vi "Handle Error.vi"(8 "error in (no error)":errorcluster, 11 "Measurement in":refnum<class "Measurement.lvclass">) -> (0 "error out":errorcluster, 2 "stop actor?":bool=TRUE, 3 "Measurement out":refnum<class "Measurement.lvclass">)   [LabVIEW 2015, in "Measurement Actor.lvlib" / "Measurement.lvclass"]
doc: "(<B>Filename</B>: Actor Framework.lvlib:Actor.lvclass:Handle Error.vi)\n\nDefines how the actor handles an error that occurred while processing a message.\n\nBy default, this method does nothing except stop the actor. This method also treats error code 43 (coming from <B>error in</B>) as a sign that the actor shut down normally. In this situation, the Handle Error method does not return the error on <B>error out</B>, meaning the actor's caller will not receive it. All other error codes will be returned on <B>error out</B>.\n\nA descendant class may override this method to change this behavior."
uses:
  Measurement.lvclass
  <vilib>/ActorFramework/Actor/Actor.lvclass/Actor.ctl
  <vilib>/ActorFramework/Actor/Actor.lvclass
  Controller/Messages/Log Status/Log Status.lvclass
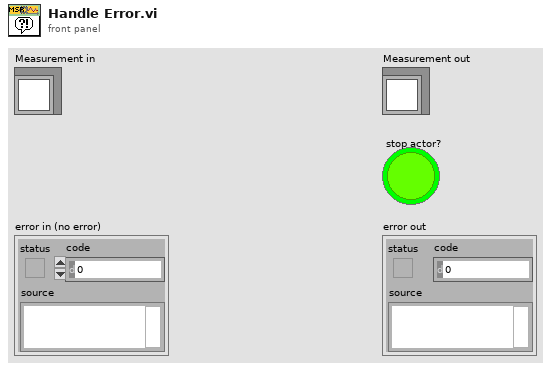
[diagram p1: front panel]
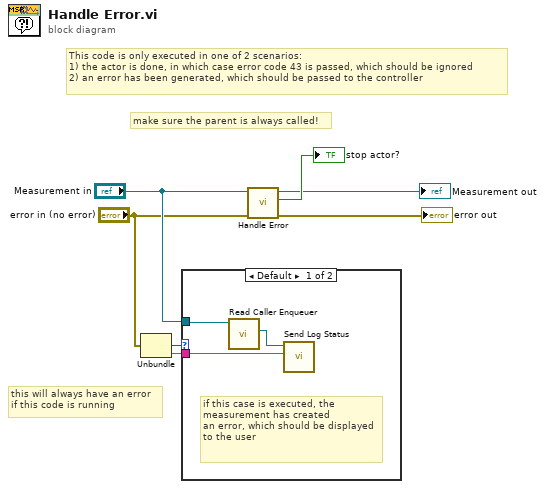
[diagram p0: block diagram]
diagram:
  # "make sure the parent is always called!"
  # "this will always have an error\nif this code is running"
  # "This code is only executed in one of 2 scenarios:\n1) the actor is done, in which case error code 43 is passed, which should be ignored\n2) an error has been generated, which should be passed to the controller"
  n1 = Unbundle("error in (no error)") -> ("code"=w2:i32, "source"=w1:string)  [unwired: 1 out]
  n2 = case shown="Default" w2 {
    tunnel: "Measurement in" -> [w9 _]
    tunnel: w1 -> [w8 _]
    frame Default {
      # "if this case is executed, the measurement has created\nan error, which should be displayed to the user"
      n3 = call <vilib>:"Read Caller Enqueuer.vi"("Actor"=w9) -> ("Caller Enqueuer"=w10:refnum<class "Message Enqueuer.lvclass">)  [unwired: 10 in]
      n4 = call "Send Log Status.vi"("String"=w8, "Message Enqueuer in"=w10) -> ()  [unwired: 8 in, 2 out]
    }
    frame 43 {
      # "\"Cancel Error\" means stop, but \"No Error\" to caller."
    }
  }
  n5 = call-parent "Handle Error.vi"("error in (no error)"="error in (no error)", "Actor in"="Measurement in") -> ("error out"=→"error out":errorcluster, "stop actor?"=→"stop actor?":bool, "Actor out"=→"Measurement out":refnum<class "Measurement.lvclass">)  [unwired: 7 in]
